vi "Read Numeric A.vi"(8 "error in (no error)":errorcluster, 11 "Divide_Int in":refnum<class "Divide_INT.lvclass">) -> (0 "error out":errorcluster, 2 "Abs_Integer.lvclass":refnum<class "Abs_Integer.lvclass">, 3 "Divide_Int out":refnum<class "Divide_INT.lvclass">)   [LabVIEW 2021, in "Divide_INT.lvclass"]
uses:
  Divide_INT.lvclass
  Abs_Types/Integer/Abs_Integer.lvclass
  Divide_INT.lvclass/Divide_INT.ctl
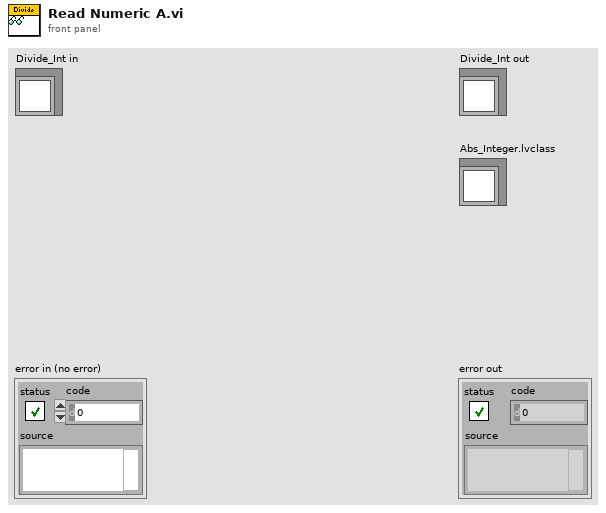
[diagram p1: front panel]
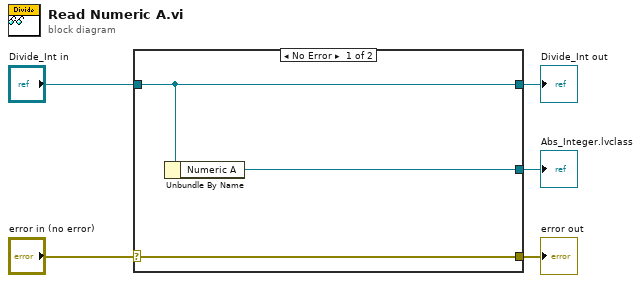
[diagram p0: block diagram]
diagram:
  n1 = case shown="No Error" "error in (no error)" {
    selector: "error in (no error)" -> [w8 w9]
    tunnel: [w8 w9] -> w4
    tunnel: [w7 w10] -> w2
    tunnel: "Divide_Int in" -> [w7 w10]
    tunnel: [w6 _] -> w1
    frame No Error {
      n2 = Unbundle By Name(w7) -> ("Numeric A"=w6:refnum<class "Abs_Integer.lvclass">)
    }
    frame Error {
    }
  }
  "error out" <- w4
  "Divide_Int out" <- w2
  "Abs_Integer.lvclass" <- w1
